vi "Read_GeneralAutoData.vi"(8 "error in (no error)":errorcluster, 11 "DriveAuto in":refnum<class "DriveAuto.lvclass">) -> (0 "error out":errorcluster, 2 "General Auto Data":T1, 3 "DriveAuto out":refnum<class "DriveAuto.lvclass">)   [LabVIEW 2017]
uses:
  DriveAuto.lvclass
  GeneralAutoData.ctl
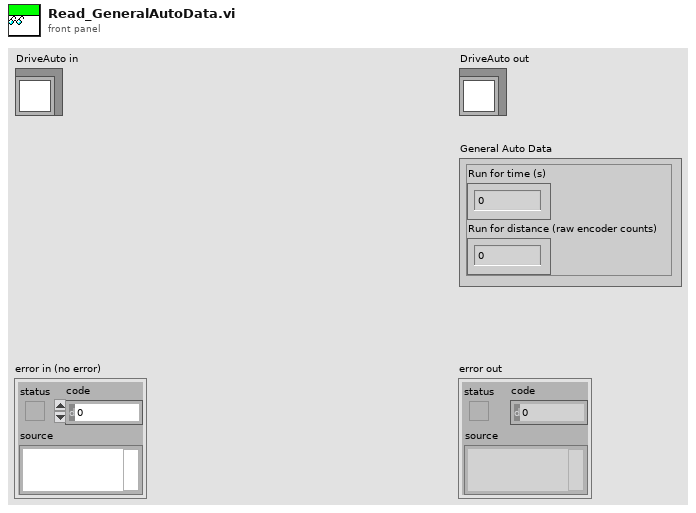
[diagram p1: front panel]
types:
  T1 = typedef "GeneralAutoData.ctl" = cluster{"Run for time (s)":dbl, "Run for distance (raw encoder counts)":dbl}
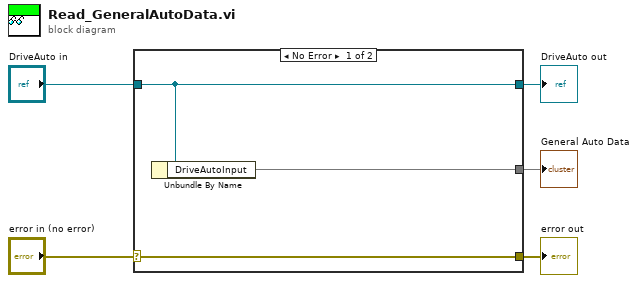
[diagram p0: block diagram]
diagram:
  n1 = case shown="No Error" "error in (no error)" {
    selector: "error in (no error)" -> [w8 w9]
    tunnel: [w8 w9] -> w4
    tunnel: [w7 w10] -> w2
    tunnel: "DriveAuto in" -> [w7 w10]
    tunnel: [w6 _] -> w1
    frame No Error {
      n2 = Unbundle By Name(w7) -> ("DriveAutoInput"=w6)
    }
    frame Error {
    }
  }
  "error out" <- w4
  "DriveAuto out" <- w2
  "General Auto Data" <- w1
